vi "HapticSTM_flt.vi"() -> ()   [LabVIEW 2019]
uses:
  <vilib>/sound2/lvsound2.llb/Sampling Mode.ctl
  <vilib>/sound2/lvsound2.llb/Sound Data Format.ctl
  SubVIs/GlobalClicksHeight_flt.vi
  <vilib>/sound2/lvsound2.llb/Sound Output Set Volume (Single).vi
  <vilib>/sound2/lvsound2.llb/Sound Output Write (DBL Single).vi
  <vilib>/Utility/file.llb/Read Delimited Spreadsheet (DBL).vi
  <userlib>/HapticSTM/HapticSTM.lvlib
  <vilib>/ptbypt/NI_PtbyPt.lvlib
panel:
  out "x/y 2":dbl
  out "x/y":dbl
  in  "Max Force":dbl=3.0 format="%.1f"
  out "ms/loop":u32=30
  in  "Sound\nActivation":bool=TRUE
  in  "Sensitivity":dbl=1.0 format="%.1f"
  in  "Volume":dbl(slide)=50.0 scale=0.0..100.0
  in  "Device ID":u32
  in  "Tab Control":T1(tab)
  in  "Surface Shift (mm)":dbl format="%.1f"
  in  "Scaling?":bool
  in  "Initial Height":dbl=70.0
  in  "Setpoint (pA)":dbl=100.0
  out "Setpoint (pA)":dbl
  in  "Maximum (pA)":dbl=7000.0
  out "Filtered Current (pA)":dbl format="%.1f"
  out "Current (pA)":dbl format="%.1f"
  out "Oy":dbl
  out "Ox":dbl
  out "W":dbl
  out "H":dbl
  out "Z Write":dbl format="%^.1e"
  out "Z Read":dbl format="%^#.1e"
  in  "Planing?":bool
  in  "Plunge Depth (pA)":dbl=180.0 format="%.1f"
  out "Button":bool
  out "Vy":dbl format="%.1f"
  out "Vz":dbl format="%.1f"
  out "Vx":dbl format="%.1f"
  out "Fy":dbl format="%.1f"
  out "Fz":dbl format="%.1f"
  out "Fx":dbl format="%.1f"
  out "phi":dbl format="%.1f"
  out "psi":dbl format="%.1f"
  out "theta":dbl format="%.1f"
  out "x":dbl format="%.1f"
  out "y":dbl format="%.1f"
  out "z":dbl format="%0.1f"
  out "Height":dbl format="%^.1e"
  in  "Hardness":dbl=0.7000000000000001 format="%.1f"
  in  "Mode":u16(ring) items=["Log w/ Exp Z", "Log w/ Lin Z"]
  in  "Reset Clicks":bool
  out "Clicks":i32
  in  "STOP":bool
  in  "START":bool
  out "Seq":i32
  out "SeqString":string
  out "Raw and Scaled Z Positions":T2(graph)
  out "Scaled Force and Current":cluster{dbl, "Filtered x":dbl, dbl}(graph)
  # "Super Ultra Mega Haptic STM Controller 3000"
  # "Nanonis"
  # "Small"
  # "Large"
  # "Sound Module"
  # "Addons"
  # "Current"
  # "Frame"
  # "Z Controller"
  # "No"
  # "Yes"
  # "Haptic Pen"
  # "Position"
  # "Force"
  # "Angles"
  # "Velocity"
  # "Surface"
  # "Clicks"
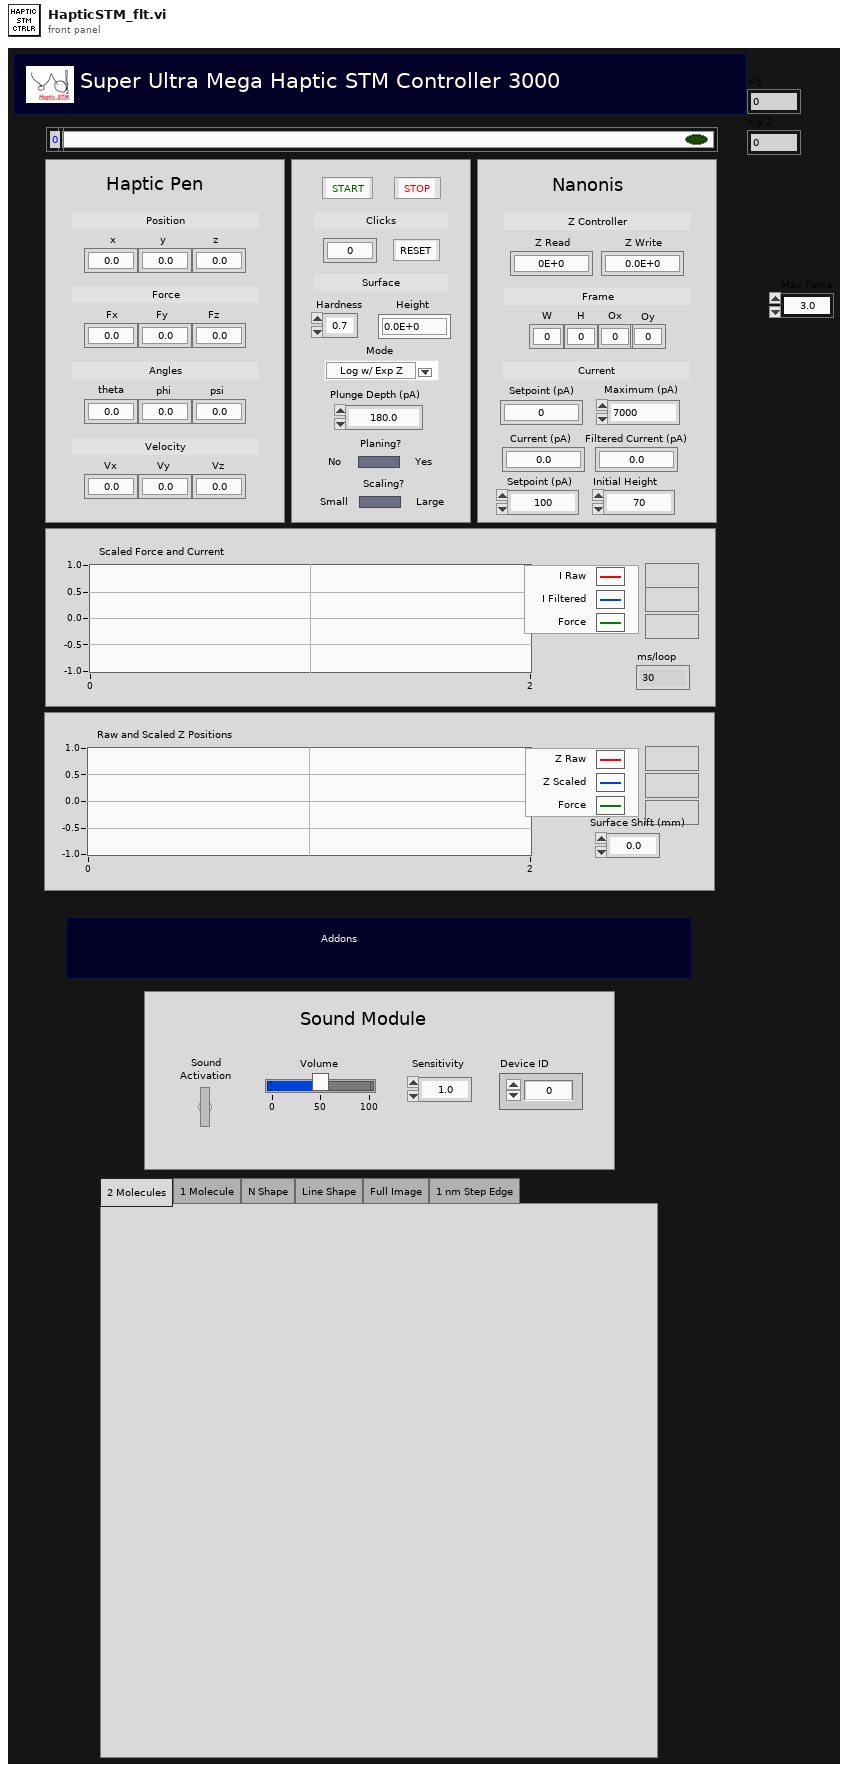
[diagram p1: front panel]
types:
  T1 = enum32{"2 Molecules", "1 Molecule", "N Shape", "Line Shape", "Full Image", "1 nm Step Edge"}
  T2 = cluster{dbl, "function return":dbl, "function return":dbl}
  T3 = typedef "Sound Data Format.ctl" = cluster{"sample rate (S/s)":dbl, "number of channels":i32, "bits per sample":i32}
  T4 = typedef "Sampling Mode.ctl" = i32
  T5 = cluster{"Current (pA)":dbl, "Filtered Current (pA)":dbl, dbl}
  T6 = typedef "Sound Output Task ID.ctl" = u32
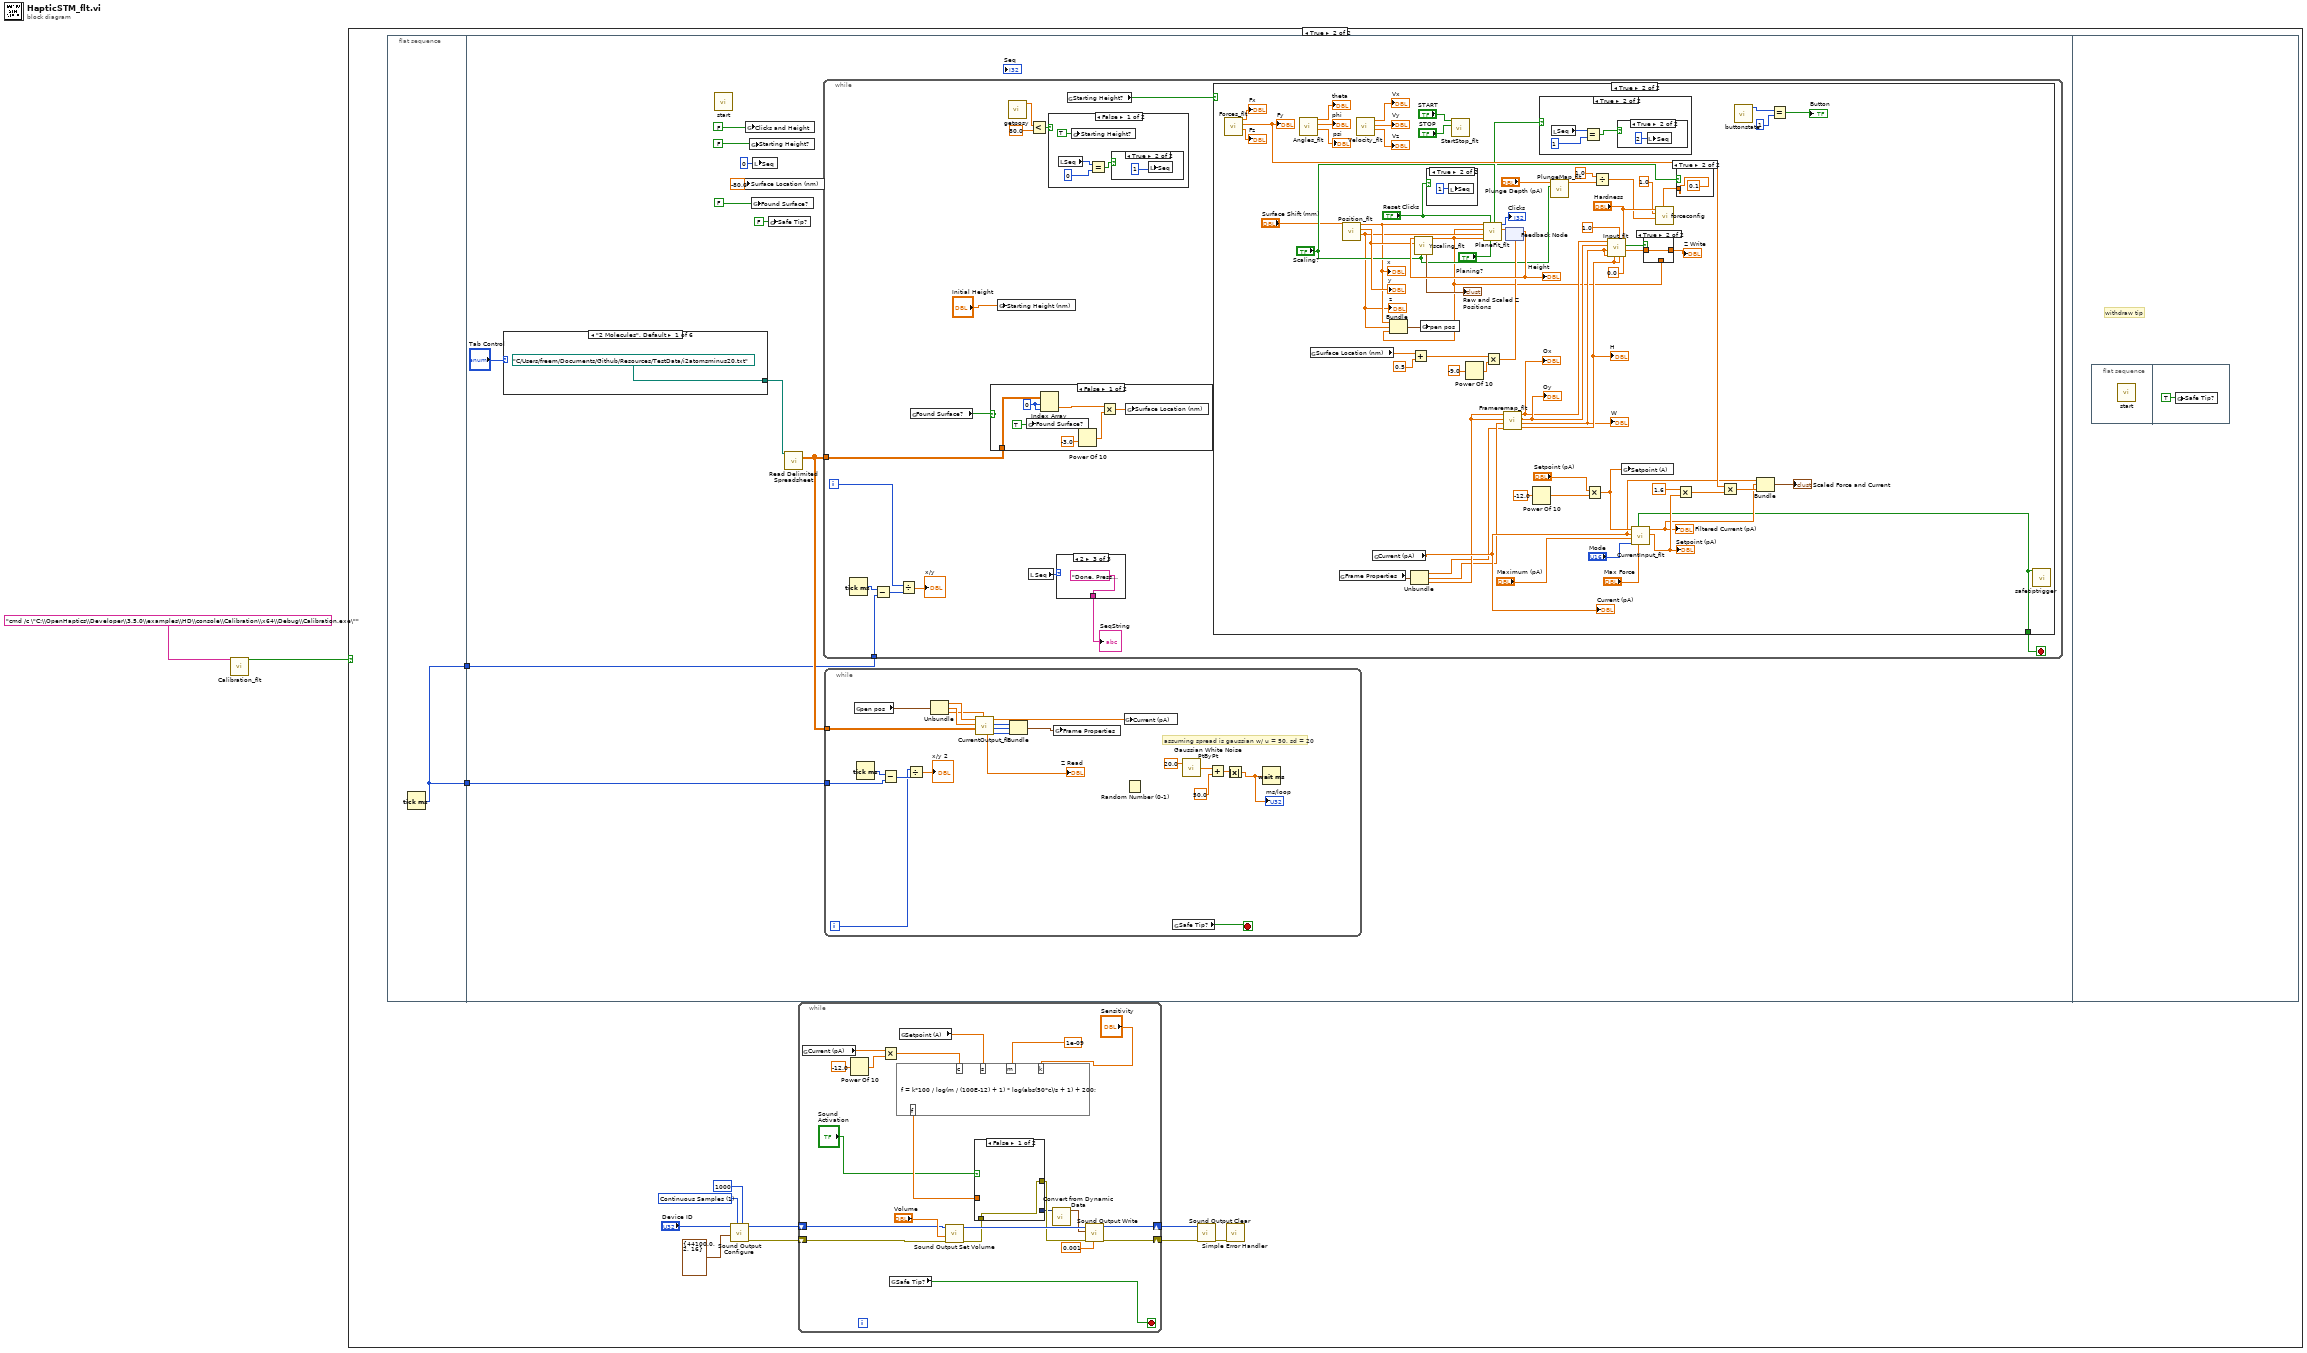
[diagram p0: block diagram]
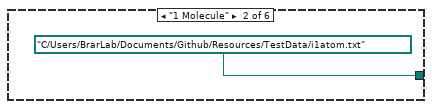
[diagram p3: hidden frame]
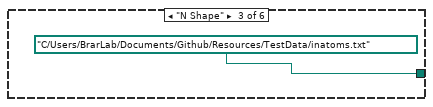
[diagram p4: hidden frame]
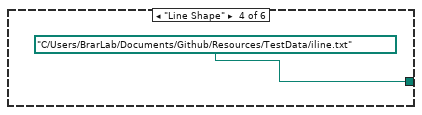
[diagram p5: hidden frame]
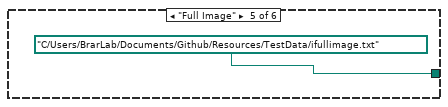
[diagram p6: hidden frame]
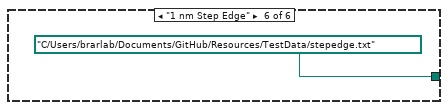
[diagram p7: hidden frame]
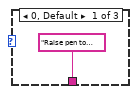
[diagram p9: hidden frame]
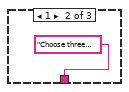
[diagram p10: hidden frame]
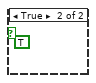
[diagram p12: hidden frame]
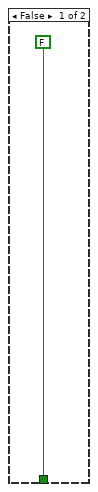
[diagram p13: hidden frame]
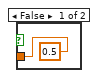
[diagram p14: hidden frame]
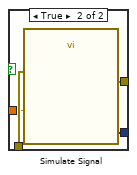
[diagram p19: hidden frame]
diagram:
  n1 = call "Calibration_flt.vi"("command line"="cmd /c \"C:\\OpenHaptics\\Developer\\3.5.0\\examples\\HD\\console\\Calibration\\x64\\Debug\\Calibration.exe\"") -> ("Calibration Complete?"=w2:bool)  [unwired: 10 in]
  n2 = case shown="True" w2 {
    frame False {
    }
    frame True {
      w12 = T4 1 items=["Finite Samples", "Continuous Samples"] ("sample mode")
      n3 = flat-sequence {
        tunnel: [w14] -> w4
        tunnel: [w14] -> w3
        tunnel: w4 -> [w16]
        tunnel: w3 -> [w15]
        frame #0 {
          n4 = Tick Count (ms)() -> (millisecond timer value=w14:u32)
        }
        frame #1 {
          n5 = case shown="\"2 Molecules\", Default" "Tab Control" {
            tunnel: [path "C:/Users/freem/Documents/Github/Resources/TestData/i2atomsminus20.txt" ("file path (dialog if empty)") path "C:/Users/BrarLab/Documents/Github/Resources/TestData/i1atom.txt" ("file path (dialog if empty)") path "C:/Users/BrarLab/Documents/Github/Resources/TestData/inatoms.txt" ("file path (dialog if empty)") path "C:/Users/BrarLab/Documents/Github/Resources/TestData/iline.txt" ("file path (dialog if empty)") path "C:/Users/BrarLab/Documents/Github/Resources/TestData/ifullimage.txt" ("file path (dialog if empty)") path "C:/Users/brarlab/Documents/GitHub/Resources/TestData/stepedge.txt" ("file path (dialog if empty)")] -> w21
            frame "2 Molecules", Default {
            }
            frame "1 Molecule" {
            }
            frame "N Shape" {
            }
            frame "Line Shape" {
            }
            frame "Full Image" {
            }
            frame "1 nm Step Edge" {
            }
          }
          n6 = call <userlib>:"start.vi"() -> ()  [unwired: 11 in, 1 out]
          n7 = global write "GlobalClicksHeight_flt.vi" "Surface Location (nm)"(-80.0 ("Surface Location")) -> ()
          n8 = global write "GlobalClicksHeight_flt.vi" "Clicks and Height"(FALSE ("Clicks and Height")) -> ()
          n9 = global write "GlobalClicksHeight_flt.vi" "Starting Height?"(FALSE ("Clicks and Height")) -> ()
          n10 = global write "GlobalClicksHeight_flt.vi" "Found Surface?"(FALSE ("Clicks and Height")) -> ()
          n11 = local write "Seq"(0 ("Seq")) -> ()
          n12 = global write "GlobalClicksHeight_flt.vi" "Safe Tip?"(FALSE ("Safe Tip?")) -> ()
          n13 = call-poly <vilib>:"Read Delimited Spreadsheet.vi"("file path (dialog if empty)"=w21) -> ("all rows"=w17:dbl[][])  [unwired: 9 in, 5 out]
          n14 = while {
            tunnel: w17 -> [w62]
            tunnel: w16 -> [w55]
            i -> [w57]
            stop <- w59 stop-if-true
            n15 = Tick Count (ms)() -> (millisecond timer value=w58:u32)
            n16 = Subtract(x=w58, y=w55) -> (x-y=w56:u32)
            n17 = Divide(x=w57, y=w56) -> (x/y=→"x/y":dbl)
            n18 = global read "GlobalClicksHeight_flt.vi" "Found Surface?"() -> (w61:bool)
            n19 = case shown="False" w61 {
              tunnel: w62 -> [w73 _]
              frame False {
                w75 = 0 ("index (row)")
                n20 = global write "GlobalClicksHeight_flt.vi" "Found Surface?"(TRUE ("Found Surface?")) -> ()
                n21 = Index Array(array=w73, index (row)=w75, index (col)=w75) -> (element=w72:dbl)
                n22 = Power Of 10(x=-3.0) -> (10^x=w70:dbl)
                n23 = Multiply(x=w72, y=w70) -> (x*y=w71:dbl)
                n24 = global write "GlobalClicksHeight_flt.vi" "Surface Location (nm)"(w71) -> ()
              }
              frame True {
              }
            }
            n25 = global write "GlobalClicksHeight_flt.vi" "Starting Height (nm)"("Initial Height") -> ()
            n26 = call <userlib>:"getposy.vi"() -> ("function return"=w68:dbl)  [unwired: 11 in]
            n27 = local read "Seq"() -> (w64:i32)
            n28 = Less?(x=w68, y=80.0) -> (x < y?=w66:bool)
            n29 = case shown="False" w66 {
              frame False {
                n30 = local read "Seq"() -> (w81:i32)
                n31 = global write "GlobalClicksHeight_flt.vi" "Starting Height?"(TRUE ("Starting Height?")) -> ()
                n32 = Equal?(x=w81, y=0) -> (x = y?=w79:bool)
                n33 = case shown="True" w79 {
                  frame False {
                  }
                  frame True {
                    n34 = local write "Seq"(1 ("Seq")) -> ()
                  }
                }
              }
              frame True {
                (unwired) TRUE ("Clicks and Height")
              }
            }
            n35 = case shown="2" w64 {
              tunnel: ["Raise pen to begin." "Choose three points, then raise the arm to plane." "Done. Press 'STOP' to stop at anytime."] -> w63
              frame 0, Default {
              }
              frame 1 {
              }
              frame 2 {
              }
            }
            "SeqString" <- w63
            n36 = global read "GlobalClicksHeight_flt.vi" "Starting Height?"() -> (w65:bool)
            n37 = case shown="True" w65 {
              tunnel: [FALSE ("Current Maxed?") w96] -> w59
              frame False {
              }
              frame True {
                n38 = call "Forces_flt.vi"() -> ("Fz"=→"Fz":dbl, "Fy"=w136:dbl, "Fx"=→"Fx":dbl)  [unwired: 9 in]
                "Fy" <- w136
                n39 = call "Angles_flt.vi"() -> ("psi"=→"psi":dbl, "phi"=→"phi":dbl, "theta"=→"theta":dbl)  [unwired: 9 in]
                n40 = global read "GlobalClicksHeight_flt.vi" "Surface Location (nm)"() -> (w105:dbl)
                n41 = global read "GlobalClicksHeight_flt.vi" "Frame Properties"() -> (w89:cluster{"FH":dbl, "FW":dbl, "Origin":dbl})
                n42 = call "Position_flt.vi"("Shift"="Surface Shift (mm)") -> ("Z"=w93:dbl, "Y"=w132:dbl, "X"=w94:dbl)  [unwired: 8 in]
                "x" <- w94
                "y" <- w132
                "z" <- w93
                n43 = call "Velocity_flt.vi"() -> ("VZ"=→"Vz":dbl, "VY"=→"Vy":dbl, "VX"=→"Vx":dbl)  [unwired: 9 in]
                n44 = global read "GlobalClicksHeight_flt.vi" "Current (pA)"() -> (w91:dbl)
                "Current (pA)" <- w91
                n45 = Unbundle(w89) -> ("FH"=w86:dbl, "FW"=w87:dbl, "Origin"=w88:dbl)
                n46 = Add(x=w105, y=0.5) -> (x+y=w102:dbl)
                n47 = case shown="True" "Reset Clicks" {
                  frame False {
                  }
                  frame True {
                    n48 = local write "Seq"(1 ("Seq")) -> ()
                  }
                }
                n49 = call "StartStop_flt.vi"("STOP"="STOP", "START"="START") -> ()  [unwired: 10 in]
                n50 = Power Of 10(x=-9.0) -> (10^x=w101:dbl)
                n51 = Multiply(x=w102, y=w101) -> (x*y=w103:dbl)
                n52 = call "Frameremap_flt.vi"("FH"=w86, "FW"=w87, "FO Z"=w88, "FO X"=w88) -> ("FH"=w116:dbl, "FW"=w115:dbl, "Z Origin"=w114:dbl, "X Origin"=w113:dbl)  [unwired: 4 in]
                "H" <- w116
                "W" <- w115
                "Ox" <- w113
                "Oy" <- w114
                n53 = feedback #1(w103) -> (w141:dbl)
                "Height" <- w141
                n54 = call "Yscaling_flt.vi"("Scaling?"="Scaling?", "Y"=w132, "Plane Height"=w141) -> ("y scaled"=w92:dbl, "output cluster"=→"Raw and Scaled Z Positions":T2)  [unwired: 7 in]
                n55 = Bundle("X"=w94, "Z"=w93, "y scaled"=w92) -> (w90:cluster{"X":dbl, "Z":dbl, "y scaled":dbl})  [unwired: 1 in]
                n56 = global write "GlobalClicksHeight_flt.vi" "pen pos"(w90) -> ()
                n57 = call "PlaneFit_flt.vi"("Planing y/n?"="Planing?", "Reset Clicks"="Reset Clicks", "Y PEN"=w92, "Z"=w93, "Nano Z"=w92, "X"=w94) -> ("Plane Height (m)"=w142:dbl, "Clicks"=→"Clicks":i32, "Planing Done?"=w125:bool)  [unwired: 3 in]
                n58 = feedback-in #1(w142) -> ()
                n59 = Power Of 10(x=-12.0) -> (10^x=w140:dbl)
                n60 = case shown="True" w125 {
                  frame False {
                  }
                  frame True {
                    n61 = local read "Seq"() -> (w161:i32)
                    n62 = Equal?(x=w161, y=1) -> (x = y?=w159:bool)
                    n63 = case shown="True" w159 {
                      frame False {
                      }
                      frame True {
                        n64 = local write "Seq"(2 ("Seq")) -> ()
                      }
                    }
                  }
                }
                n65 = call "PlungeMap_flt.vi"("Scaling?"="Scaling?", "Input (pA)"="Plunge Depth (pA)") -> ("output"=w106:dbl)  [unwired: 9 in]
                n66 = Multiply(x="Setpoint (pA)", y=w140) -> (x*y=w111:dbl)
                n67 = Divide(x=1.0, y=w106) -> (x/y=w117:dbl)
                n68 = call "Input_flt.vi"("Current * 10^input"=0.0, "Sensitivity"="Hardness", "Scopez"=w116, "Drag"=1.0, "FH"=w116, "FW"=w115, "Scopex"=w115, "Z origin"=w114, "X origin"=w113) -> ("Scaled Current"=w119:dbl, "feedback"=w121:bool)  [unwired: 1 in]
                n69 = global write "GlobalClicksHeight_flt.vi" "Setpoint (A)"(w111) -> ()
                n70 = call "CurrentInput_flt.vi"("maxforcey"="Max Force", "Mode"="Mode", "Maximum (pA)"="Maximum (pA)", "Current (pA)"=w91, "Setpoint (A)"=w111) -> ("Setpoint (pA)"=w108:dbl, "Filtered Current (pA)"=w99:dbl, "Safetip?"=w96:bool)  [unwired: 4 in]
                "Filtered Current (pA)" <- w99
                "Setpoint (pA)" <- w108
                n71 = case shown="True" w121 {
                  tunnel: [w156 w157] -> w120
                  tunnel: w119 -> [_ w157]
                  tunnel: w92 -> [w156 _]
                  frame False {
                  }
                  frame True {
                  }
                }
                "Z Write" <- w120
                n72 = case shown="True" "Scaling?" {
                  tunnel: [0.5 0.1] -> w98
                  frame False {
                  }
                  frame True {
                  }
                }
                n73 = call <userlib>:"forceconfig.vi"("spc"=w98, "c"=w117, "b"=1.0, "a"="Hardness") -> ()  [unwired: 8 in]
                n74 = Multiply(x=1.6 ("y"), y=w108) -> (x*y=w133:dbl)
                n75 = Multiply(x=w136, y=w133) -> (x*y=w135:dbl)
                n76 = call <userlib>:"buttonstate.vi"() -> ("function return"=w131:i32)  [unwired: 11 in]
                n77 = Bundle("Current (pA)"=w91, "Filtered Current (pA)"=w99, w135) -> (→"Scaled Force and Current":T5)  [unwired: 1 in]
                n78 = Equal?(x=w131, y=1) -> (x = y?=→"Button":bool)
                n79 = call <userlib>:"safetiptrigger.vi"("triggered"=w96) -> ()  [unwired: 11 in]
              }
            }
          }
          n80 = while {
            tunnel: w17 -> [w46]
            tunnel: w15 -> [w27]
            i -> [w28]
            stop <- w47 stop-if-true
            # "assuming spread is gaussian w/ u = 50, sd = 20"
            n81 = global read "GlobalClicksHeight_flt.vi" "pen pos"() -> (w36:cluster{"X":dbl, "Z":dbl, "y scaled":dbl})
            n82 = Tick Count (ms)() -> (millisecond timer value=w30:u32)
            n83 = Subtract(x=w30, y=w27) -> (x-y=w29:u32)
            n84 = Divide(x=w28, y=w29) -> (x/y=→"x/y 2":dbl)
            n85 = Unbundle(w36) -> ("X"=w42:dbl, "Z"=w41:dbl, "y scaled"=w38:dbl)
            n86 = call "CurrentOutput_flt.vi"("y scaled"=w38, "array"=w46, "Z Input"=w41, "X Input"=w42) -> ("O"=w43:i32, "FW"=w44:i32, "FH"=w45:i32, "Current Out (pA)"=w39:dbl, "Zread"=→"Z Read":dbl)  [unwired: 3 in]
            n87 = Bundle("FH"=w45, "FW"=w44, "O"=w43) -> (w37:cluster{"FH":i32, "FW":i32, "O":i32})  [unwired: 1 in]
            n88 = global write "GlobalClicksHeight_flt.vi" "Frame Properties"(w37) -> ()
            n89 = global write "GlobalClicksHeight_flt.vi" "Current (pA)"(w39) -> ()
            n90 = Random Number (0-1)() -> ()  [unwired: 1 out]
            n91 = global read "GlobalClicksHeight_flt.vi" "Safe Tip?"() -> (w47:bool)
            n92 = call <vilib>:"Gaussian White Noise PtByPt.vi"("standard deviation"=20.0) -> ("Gaussian white noise"=w34:dbl)  [unwired: 2 in]
            n93 = Add(x=w34, y=50.0) -> (x+y=w32:dbl)
            n94 = Absolute Value(x=w32) -> (abs(x)=w31:dbl)
            "ms/loop" <- w31
            n95 = Wait (ms)(milliseconds to wait=w31) -> ()  [unwired: 1 out]
          }
        }
        frame #2 {
          # "withdraw tip"
          n96 = flat-sequence {
            frame #0 {
              n97 = call <userlib>:"start.vi"() -> ()  [unwired: 11 in, 1 out]
            }
            frame #1 {
              n98 = global write "GlobalClicksHeight_flt.vi" "Safe Tip?"(TRUE ("Safe Tip?")) -> ()
            }
          }
        }
      }
      n99 = call <vilib>:"Sound Output Configure.vi"("number of samples/ch"=1000 ("Number of Samples/ch"), "sample mode"=w12, "sound format"=T3 {"sample rate (S/s)"=44100.0, "number of channels"=2, "bits per sample"=16} ("Sound Format"), "device ID"="Device ID") -> ("error out"=w8:errorcluster, "task ID"=w9:T6)  [unwired: 6 in]
      n100 = while {
        shift-right: [w176] -> w7
        shift-left: w9 -> [w178]
        shift-right: [w175] -> w6
        shift-left: w8 -> [w177]
        stop <- w165 stop-if-true
        n101 = global read "GlobalClicksHeight_flt.vi" "Current (pA)"() -> (w168:dbl)
        n102 = Power Of 10(x=-12.0) -> (10^x=w170:dbl)
        n103 = Multiply(x=w168, y=w170) -> (x*y=w167:dbl)
        n104 = global read "GlobalClicksHeight_flt.vi" "Safe Tip?"() -> (w165:bool)
        n105 = global read "GlobalClicksHeight_flt.vi" "Setpoint (A)"() -> (w172:dbl)
        n106 = formula code="f = k*100 / log(m / (100E-12) + 1) * log(abs(50*c)/s + 1) + 200;"("c"=w167, "m"=1e-09 ("input variable"), "s"=w172, "k"="Sensitivity") -> ("f"=w171:dbl)
        n107 = call-poly <vilib>:"Sound Output Set Volume.vi"("error in (no error)"=w177, "volume"="Volume", "task ID"=w178) -> ("error out"=w181:errorcluster, "task ID out"=w184:T6)  [unwired: 7 in]
        n108 = case shown="False" "Sound\nActivation" {
          tunnel: w181 -> [w185 w189]
          tunnel: [w185 w188] -> w180
          tunnel: [_ w187] -> w179
          tunnel: w171 -> [_ w186]
          frame False {
          }
          frame True {
            n109 = call "Simulate Signal"("Frequency"=w186, "error in (no error)"=w189) -> ("Sine"=w187:dynamicdata, "error out"=w188:errorcluster)  [unwired: 12 in]
          }
        }
        n110 = call "Convert from Dynamic Data"("Dynamic Data Type"=w179) -> ("Waveform"=w182:waveform(dbl))  [unwired: 3 in]
        n111 = call-poly <vilib>:"Sound Output Write.vi"("timeout (sec)"=0.001, "error in (no error)"=w180, "data"=w182, "task ID"=w184) -> ("error out"=w175:errorcluster, "task ID out"=w176:T6)  [unwired: 6 in]
      }
      n112 = call <vilib>:"Sound Output Clear.vi"("error in (no error)"=w6, "task ID"=w7) -> ("error out"=w11:errorcluster)  [unwired: 9 in]
      n113 = call <vilib>:"Simple Error Handler.vi"("error in (no error)"=w11) -> ()  [unwired: 4 in, 5 out]
    }
  }
